vi "circleBox.vi"(1 "Circles 3":T2(array[cluster])) -> (0 "output cluster":T1)   [LabVIEW 2023]
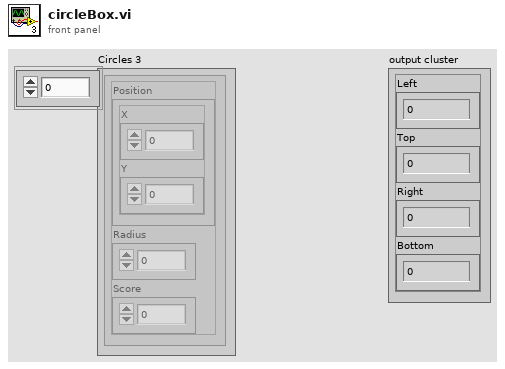
[diagram p1: front panel]
types:
  T1 = cluster{"Left":i32, "Top":i32, "Right":i32, "Bottom":i32}
  T2 = cluster{"Position":cluster{"X":sgl, "Y":sgl}, "Radius":dbl, "Score":dbl}[]
  T3 = cluster{"Position":cluster{"X":sgl, "Y":sgl}, "Radius":dbl, "Score":dbl}
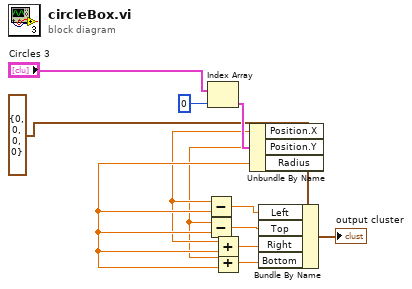
[diagram p0: block diagram]
diagram:
  n1 = Index Array(array="Circles 3", index=0) -> (element=w11:T3)
  n2 = Unbundle By Name(w11) -> ("Position.X"=w2:sgl, "Position.Y"=w1:sgl, "Radius"=w3:dbl)
  n3 = Subtract(x=w2, y=w3) -> (x-y=w5:dbl)
  n4 = Subtract(x=w1, y=w3) -> (x-y=w4:dbl)
  n5 = Add(x=w2, y=w3) -> (x+y=w8:dbl)
  n6 = Add(x=w1, y=w3) -> (x+y=w9:dbl)
  n7 = Bundle By Name(cluster=T1 {"Left"=0, "Top"=0, "Right"=0, "Bottom"=0} ("Rectangle"), "Left"=w5, "Top"=w4, "Right"=w8, "Bottom"=w9) -> (→"output cluster":T1)
